vi "update_polarization.vi"(0 "Iterations per time step":i32, 1 "Pn in":dbl, 2 "Pe in":dbl, 3 "T1e (s)":dbl, 4 "T1n (s)":dbl, 5 "Alpha":dbl, 6 "Beta":dbl, 7 "C":dbl) -> (20 "Pn out":dbl, 27 "Pe out":dbl)   [LabVIEW 2015]
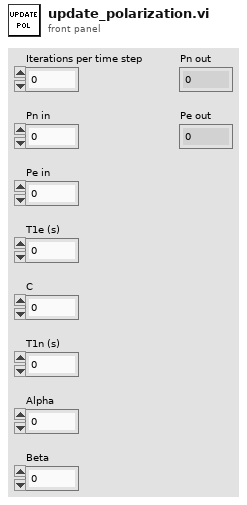
[diagram p1: front panel]
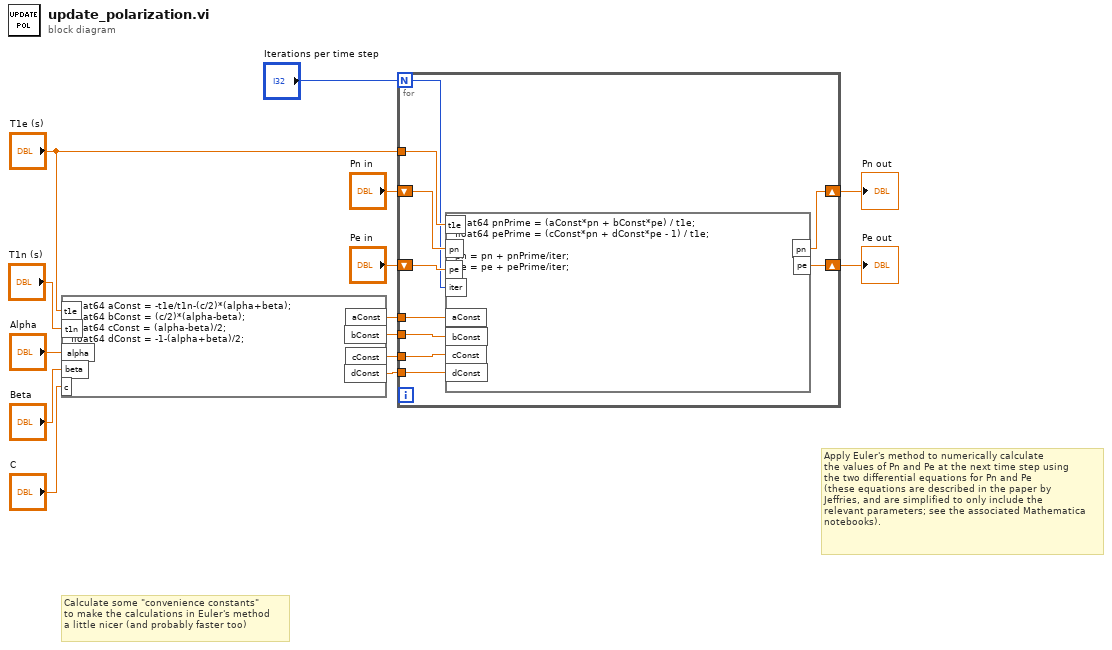
[diagram p0: block diagram]
diagram:
  # "Apply Euler's method to numerically calculate\nthe values of Pn and Pe at the next time step using\nthe two differential equations for Pn and Pe\n(these equations are described in the paper by\nJeffries, and are simplified to only include the\nrelevant parameters; see the associated Mathematica\nnotebooks)."
  # "Calculate some \"convenience constants\"\nto make the calculations in Euler's method\na little nicer (and probably faster too)"
  n1 = formula code="float64 aConst = -t1e/t1n-(c/2)*(alpha+beta);\nfloat64 bConst = (c/2)*(alpha-beta);\nfloat64 cConst = (alpha-beta)/2;\nfloat64 dConst = -1-(alpha+beta)/2;"("t1e"="T1e (s)", "t1n"="T1n (s)", "alpha"="Alpha", "beta"="Beta", "c"="C") -> ("aConst"=w8:dbl, "bConst"=w9:dbl, "cConst"=w10:dbl, "dConst"=w11:dbl)
  n2 = for {
    N: "Iterations per time step" -> [w17]
    shift-right: [w16] -> w13
    shift-left: "Pn in" -> [w20]
    shift-right: [w15] -> w14
    shift-left: "Pe in" -> [w19]
    tunnel: w8 -> [w24]
    tunnel: w9 -> [w23]
    tunnel: w10 -> [w22]
    tunnel: w11 -> [w21]
    tunnel: "T1e (s)" -> [w18]
    n3 = formula code="float64 pnPrime = (aConst*pn + bConst*pe) / t1e;\nfloat64 pePrime = (cConst*pn + dConst*pe - 1) / t1e;\n\npn = pn + pnPrime/iter;\npe = pe + pePrime/iter;"("pn"=w20, "pe"=w19, "t1e"=w18, "aConst"=w24, "bConst"=w23, "cConst"=w22, "dConst"=w21, "iter"=w17) -> ("pn"=w16:dbl, "pe"=w15:dbl)
  }
  "Pe out" <- w14
  "Pn out" <- w13
